vi "openCommunication.vi"(8 "error in (no error)":errorcluster, 11 "ESP8266 in":refnum<class "ESP8266.lvclass">) -> (0 "error out":errorcluster, 3 "ESP8266 out":refnum<class "ESP8266.lvclass">)   [LabVIEW 2020, in "ESP8266.lvclass"]
uses:
  ESP8266.lvclass
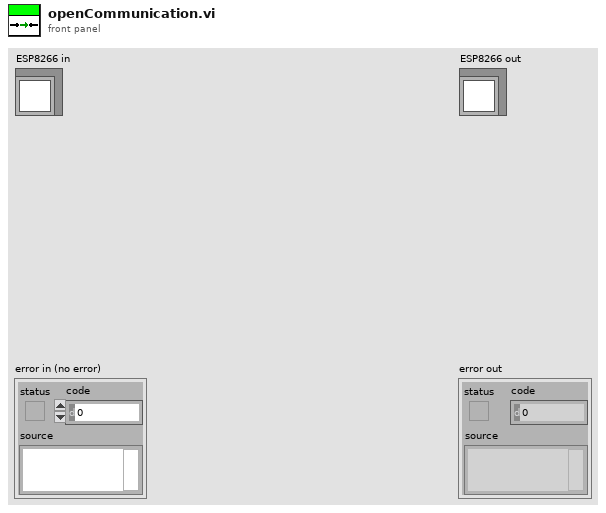
[diagram p1: front panel]
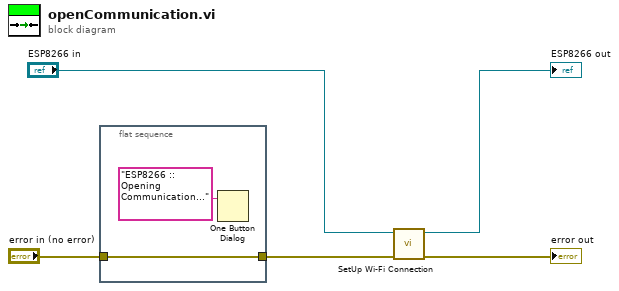
[diagram p0: block diagram]
diagram:
  n1 = flat-sequence {
    tunnel: "error in (no error)" -> [w6]
    tunnel: [w6] -> w1
    frame #0 {
      n2 = One Button Dialog(message="ESP8266 :: Opening Communication...") -> ()  [unwired: 1 in, 1 out]
    }
  }
  n3 = call-dynamic "SetUp Wi-Fi Connection.vi"("error in (no error)"=w1, "ESP8266 in"="ESP8266 in") -> ("error out"=→"error out":errorcluster, "ESP8266 out"=→"ESP8266 out":refnum<class "ESP8266.lvclass">)  [unwired: 8 in]
